vi "Write Mode.vi"(5 "Username":string, 6 "Password":string, 7 "Address":string, 8 "Error In":errorcluster) -> (0 "Error Out":errorcluster)   [LabVIEW 2018, in "Tests.lvlib" / "Channel.lvlib"]
uses:
  Channel.lvlib
  src/Toolkit/Channel/Typedefs/Modes.ctl
  src/Toolkit/Channel/Channel.lvclass/Channel.ctl
  src/Toolkit/Session/Session.lvclass/Session.ctl
  src/Toolkit/SSH/SSH.lvclass/SSH.ctl
  src/Toolkit/Session/Utility/Read Shared Library.vi
  src/Toolkit/SSH/Utility/Read Shared Library.vi
  src/Toolkit/Support/Check Status.vi
  <vilib>/addons/_JKI Toolkits/Caraya/classes/Test/Test.lvclass
  <vilib>/addons/_JKI Toolkits/Caraya/classes/Assert/Assert.lvclass
  src/Toolkit/Channel/Channel.lvclass
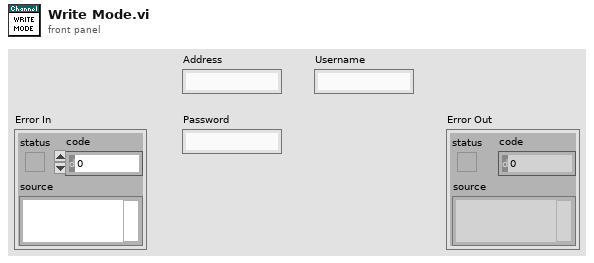
[diagram p1: front panel]
types:
  T1 = typedef "Toolkit.lvlib/Channel.lvclass/Modes.ctl" = i32
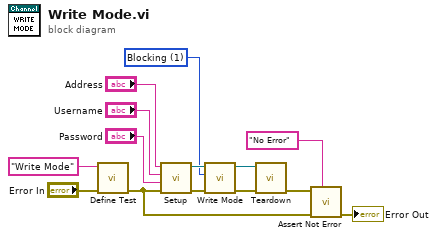
[diagram p0: block diagram]
diagram:
  w1 = T1 1 items=["Non-Blocking", "Blocking"] ("Mode")
  n1 = call <vilib>:"Define Test.vi"("error in (no error)"="Error In", "Label (VI Title)"="Write Mode") -> ("error out"=w11:errorcluster)  [unwired: 9 in]
  n2 = call "Setup.vi"("Error In"=w11, "Password"="Password", "Username"="Username", "Address"="Address") -> ("Error Out"=w2:errorcluster, "Channel"=w5:refnum<class "Channel.lvclass">)  [unwired: 6 in]
  n3 = call "Write Mode.vi"("Error In"=w2, "Mode"=w1, "Channel In"=w5) -> ("Error Out"=w3:errorcluster, "Channel Out"=w4:refnum<class "Channel.lvclass">)  [unwired: 7 in]
  n4 = call "Teardown.vi"("Error In"=w3, "Channel"=w4) -> ("Error Out"=w7:errorcluster)  [unwired: 9 in]
  n5 = call <vilib>:"Assert Not Error.vi"("Label"="No Error", "error in (no error)"=w11, "Not Error?"=w7) -> ("error out"=→"Error Out":errorcluster)  [unwired: 8 in]
